vi "Write tree ref.vi"(8 "error in (no error)":errorcluster, 9 "tree ref":refnum<k24>, 11 "alias-tree in":refnum<class "alias-tree.lvclass">) -> (0 "error out":errorcluster, 3 "alias-tree out":refnum<class "alias-tree.lvclass">)   [LabVIEW 2017, in "vs-tree-utility.lvlib" / "alias-tree.lvclass"]
uses:
  alias-tree.lvclass
  NationalInstruments.VeriStand.SystemStorageUI
  alias-tree.lvclass/alias-tree.ctl
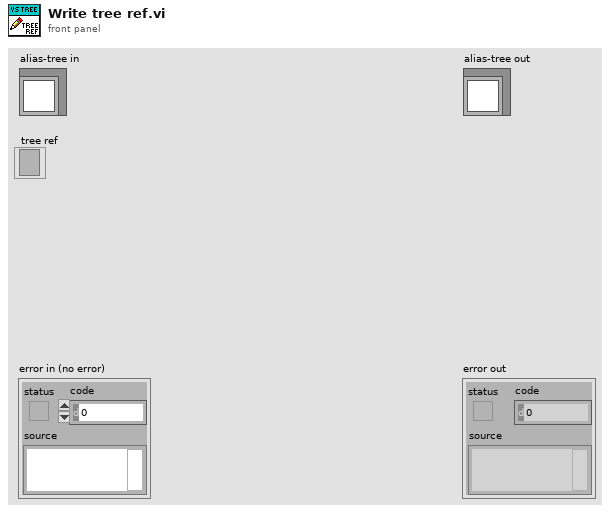
[diagram p1: front panel]
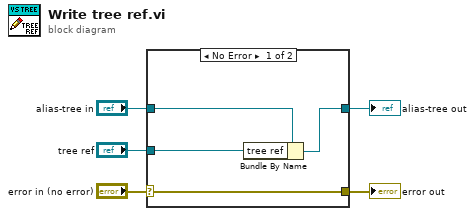
[diagram p0: block diagram]
diagram:
  n1 = case shown="No Error" "error in (no error)" {
    selector: "error in (no error)" -> [w9 w11]
    tunnel: [w9 w11] -> w4
    tunnel: [w6 w10] -> w2
    tunnel: "alias-tree in" -> [w8 w10]
    tunnel: "tree ref" -> [w7 _]
    frame No Error {
      n2 = Bundle By Name(cluster=w8, "tree ref"=w7) -> (w6:refnum<class "alias-tree.lvclass">)
    }
    frame Error {
    }
  }
  "error out" <- w4
  "alias-tree out" <- w2
